vi "InitMotionParams.vi"(8 "error in (no error)":errorcluster, 11 "Axis in":refnum<class "Axis.lvclass">) -> (0 "error out":errorcluster, 3 "Axis out":refnum<class "Axis.lvclass">)   [LabVIEW 2020, in "Axis.lvclass"]
uses:
  Axis.lvclass
  C:/Users/Jonathan/Documents/Clearpath SDK/CSharp Examples/CLRWrapper/x64/Debug/CLRWrapper.dll
  CSharp Examples/CLRWrapper/x64/Debug/CLRWrapper.dll
  Axis.lvclass/Axis.ctl
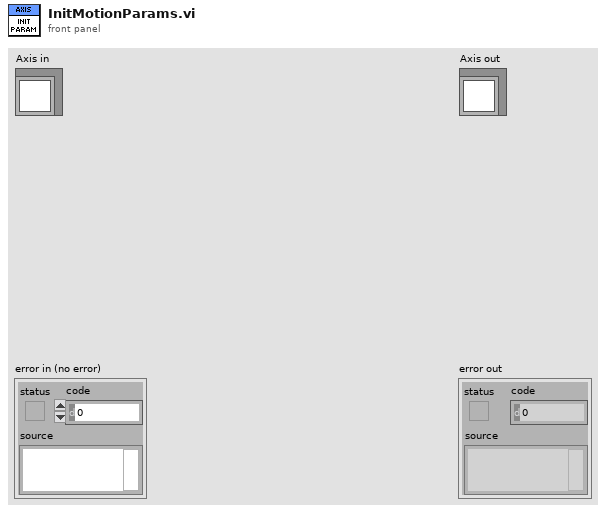
[diagram p1: front panel]
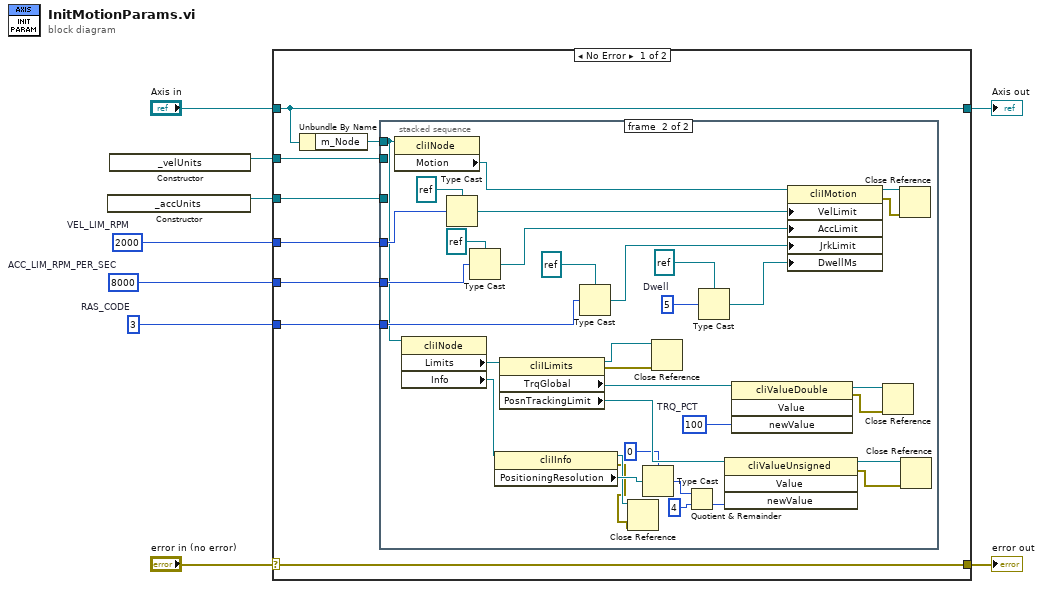
[diagram p0: block diagram]
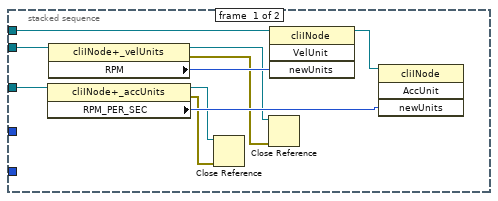
[diagram p2: hidden frame]
diagram:
  w1 = 3  # RAS_CODE
  w2 = 8000  # ACC_LIM_RPM_PER_SEC
  w3 = 2000  # VEL_LIM_RPM
  n1 = constructor class="cliINode+_accUnits"() -> (reference out=w4:refnum<k24>)  [unwired: 3 in, 2 out]
  n2 = constructor class="cliINode+_velUnits"() -> (reference out=w5:refnum<k24>)  [unwired: 3 in, 2 out]
  n3 = case shown="No Error" "error in (no error)" {
    selector: "error in (no error)" -> [w17 w63]
    tunnel: [w17 w63] -> w8
    tunnel: [w16 w62] -> w6
    tunnel: "Axis in" -> [w16 w62]
    tunnel: w5 -> [w14 _]
    tunnel: w4 -> [w13 _]
    tunnel: w3 -> [w12 _]
    tunnel: w2 -> [w11 _]
    tunnel: w1 -> [w10 _]
    frame No Error {
      n4 = Unbundle By Name(w16) -> ("m_Node"=w15:refnum<k24>)
      n5 = stacked-sequence {
        tunnel: w15 -> [w27 w53]
        tunnel: w14 -> [w26 _]
        tunnel: w13 -> [w25 _]
        tunnel: w12 -> [_ w58]
        tunnel: w11 -> [_ w56]
        tunnel: w10 -> [_ w54]
        frame #0 {
          n6 = property class="cliINode+_accUnits"(reference=w25) -> (reference out=w21:refnum<k24>, error out=w20:errorcluster, "RPM_PER_SEC"=w22:i32)  [unwired: 1 in]
          n7 = property class="cliINode+_velUnits"(reference=w26) -> (reference out=w19:refnum<k24>, error out=w18:errorcluster, "RPM"=w24:i32)  [unwired: 1 in]
          n8 = Close Reference(reference=w21, error in (no error)=w20) -> ()  [unwired: 1 out]
          n9 = Close Reference(reference=w19, error in (no error)=w18) -> ()  [unwired: 1 out]
          n10 = invoke class="cliINode" method="VelUnit"(reference=w27, "newUnits"=w24) -> (reference out=w23:refnum<k24>)  [unwired: 2 in, 3 out]
          n11 = invoke class="cliINode" method="AccUnit"(reference=w23, "newUnits"=w22) -> ()  [unwired: 2 in, 4 out]
        }
        frame #1 {
          w38 = 5  # Dwell
          w48 = u32 100  # TRQ_PCT
          n12 = property class="cliINode"(reference=w53) -> ("Motion"=w61:refnum<k24>)  [unwired: 1 in, 2 out]
          n13 = property class="cliINode"(reference=w53) -> ("Limits"=w52:refnum<k24>, "Info"=w46:refnum<k24>)  [unwired: 1 in, 2 out]
          n14 = Type Cast(type=refnum<k24> refnum ("VelLimit"), x=w58) -> (*(type *) &x=w60:refnum<k24>)
          n15 = Type Cast(type=refnum<k24> refnum ("AccLimit"), x=w56) -> (*(type *) &x=w50:refnum<k24>)
          n16 = property class="cliIInfo"(reference=w46) -> (reference out=w29:refnum<k24>, error out=w28:errorcluster, "PositioningResolution"=w44:refnum<k24>)  [unwired: 1 in]
          n17 = property class="cliILimits"(reference=w52) -> (reference out=w31:refnum<k24>, error out=w30:errorcluster, "TrqGlobal"=w51:refnum<k24>, "PosnTrackingLimit"=w47:refnum<k24>)  [unwired: 1 in]
          n18 = Type Cast(type=refnum<k24> refnum ("JrkLimit"), x=w54) -> (*(type *) &x=w49:refnum<k24>)
          n19 = Close Reference(reference=w29, error in (no error)=w28) -> ()  [unwired: 1 out]
          n20 = Type Cast(type=0, x=w44) -> (*(type *) &x=w43:i32)
          n21 = Close Reference(reference=w31, error in (no error)=w30) -> ()  [unwired: 1 out]
          n22 = Quotient & Remainder(x=w43, y=4) -> (floor(x/y)=w41:i32)  [unwired: 1 out]
          n23 = Type Cast(type=refnum<k24> refnum ("DwellMs"), x=w38) -> (*(type *) &x=w39:refnum<k24>)
          n24 = invoke class="cliValueUnsigned" method="Value"(reference=w47, "newValue"=w41) -> (reference out=w33:refnum<k24>, error out=w32:errorcluster)  [unwired: 2 in, 2 out]
          n25 = invoke class="cliValueDouble" method="Value"(reference=w51, "newValue"=w48) -> (reference out=w35:refnum<k24>, error out=w34:errorcluster)  [unwired: 2 in, 2 out]
          n26 = property class="cliIMotion"(reference=w61, "VelLimit"=w60, "AccLimit"=w50, "JrkLimit"=w49, "DwellMs"=w39) -> (reference out=w37:refnum<k24>, error out=w36:errorcluster)  [unwired: 1 in]
          n27 = Close Reference(reference=w35, error in (no error)=w34) -> ()  [unwired: 1 out]
          n28 = Close Reference(reference=w37, error in (no error)=w36) -> ()  [unwired: 1 out]
          n29 = Close Reference(reference=w33, error in (no error)=w32) -> ()  [unwired: 1 out]
        }
      }
    }
    frame Error {
    }
  }
  "error out" <- w8
  "Axis out" <- w6
